vi "ERIO RT STATE Alarm.vi"(6 "Supervisory Variables In":T4={"Alarm Threshold"=0.0, "Shutdown"=FALSE, "Enable SNS Alarm"=FALSE, "Enable SNS Stage Notification"=FALSE, "Enable SQS Notification"=FALSE, "Enable S3 TDMS Signal Capture"=FALSE, "Enable SystemLink Signal Capture"=FALSE, "Capture Signal"=FALSE, "Server Update"=FALSE, "AWS Access Key"="AKIAINLDO2Y2PDFEWDOQ", "AWS Secret Key"="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", "Phone Number"="+15037066913", "Region"=enum."us-west-2", "AWS SQS Queue"="mynicloud-demotest2", "AWS S3 Bucket"="mynicloud-demotest2"}, 7 "RT State In":T1, 8 "error in (no error)":errorcluster, 9 "AWS Variables In":T6, 11 "EEISysLink.lvclass In":refnum<class "EEISysLink.lvclass">) -> (0 "error out":errorcluster, 1 "AWS Variables Out":T6, 3 "EEISysLink.lvclass Out":refnum<class "EEISysLink.lvclass">, 4 "Supervisory Variables Out":T4={"Alarm Threshold"=0.0, "Shutdown"=FALSE, "Enable SNS Alarm"=FALSE, "Enable SNS Stage Notification"=FALSE, "Enable SQS Notification"=FALSE, "Enable S3 TDMS Signal Capture"=FALSE, "Enable SystemLink Signal Capture"=FALSE, "Capture Signal"=FALSE, "Server Update"=FALSE, "AWS Access Key"="AKIAINLDO2Y2PDFEWDOQ", "AWS Secret Key"="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", "Phone Number"="+15037066913", "Region"=enum."us-west-2", "AWS SQS Queue"="mynicloud-demotest2", "AWS S3 Bucket"="mynicloud-demotest2"}, 5 "RT State Out":T1)   [LabVIEW 2017]
doc: "Execute the alarm state. Currently that means reporting the alarm in prescribed paths. \n\nJames Tillett P.E.\nEndeavor Engineering Inc.\nwww.endeavoreng.com"
uses:
  Class EEISysLink/EEISysLink.lvclass
  Controls/ERIO AWS Toolkit Variables.ctl
  <vilib>/AWS Toolkit/SQS/Queue/Queue.lvclass
  <vilib>/AWS Toolkit/SNS/Phone Number/Phone Number.lvclass
  <vilib>/AWS Toolkit/S3/Bucket/Bucket.lvclass
  Controls/ERIO Supervisory Variables.ctl
  <vilib>/AWS Toolkit/Core/HTTP Request/Region.ctl
  Controls/ERIO RT State Variables.ctl
  Controls/ERIO SystemStates.ctl
  Controls/ERIO Queue Data.ctl
  Controls/ERIO Worker Variables.ctl
  Controls/ERIO SoundOptions.ctl
  Class EEISysLink/Controls/SL Tag Scope.ctl
  <vilib>/AWS Toolkit/Core/HTTP Request/HTTP Request.lvclass
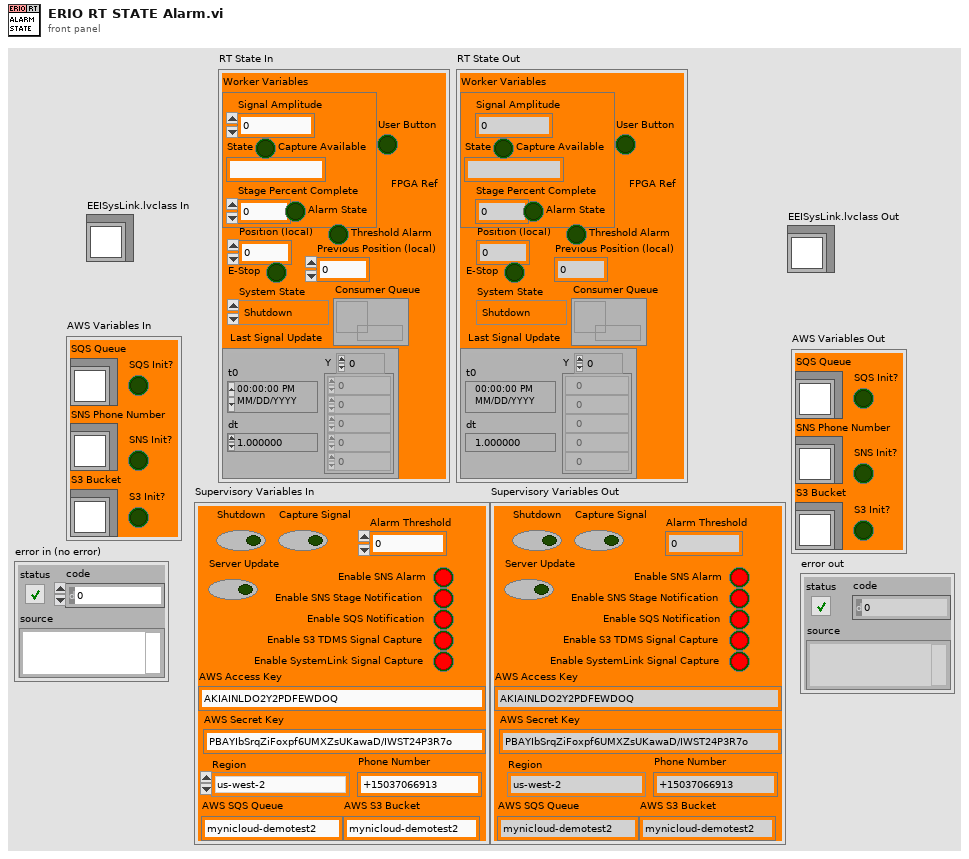
[diagram p1: front panel]
types:
  T1 = typedef "ERIO RT State Variables.ctl" = cluster{"Position (local)":i16, "E-Stop":bool, "System State":T2, "FPGA Ref":refnum<k20>, "Previous Position (local)":i16, "Consumer Queue":refnum<queue>, "Worker Variables":T3, "Threshold Alarm":bool, "User Button":bool, "Last Signal Update":waveform(dbl)}
  T2 = typedef "ERIO SystemStates.ctl" = enum16{"Shutdown", "E-STOP", "Reset Process", "Stage 1", "Stage 2", "Stage 3", "Alarm State"}
  T3 = typedef "ERIO Worker Variables.ctl" = cluster{"Signal Amplitude":dbl, "State":string, "Stage Percent Complete":dbl, "Alarm State":bool, "Capture Available":bool}
  T4 = typedef "ERIO Supervisory Variables.ctl" = cluster{"Alarm Threshold":dbl, "Shutdown":bool, "Enable SNS Alarm":bool, "Enable SNS Stage Notification":bool, "Enable SQS Notification":bool, "Enable S3 TDMS Signal Capture":bool, "Enable SystemLink Signal Capture":bool, "Capture Signal":bool, "Server Update":bool, "AWS Access Key":string, "AWS Secret Key":string, "Phone Number":string, "Region":T5, "AWS SQS Queue":string, "AWS S3 Bucket":string}
  T5 = typedef "NI_AWS_Core.lvlib/HTTP Request.lvclass/Region.ctl" = enum16{"us-east-1", "us-east-2", "us-west-1", "us-west-2", "ap-northeast-1", "ap-northeast-2", "ap-southeast-1", "ap-southeast-2", "ca-central-1", "eu-central-1", "eu-west-1", "eu-west-2", "sa-east-1"}
  T6 = typedef "ERIO AWS Toolkit Variables.ctl" = cluster{"SQS Queue":refnum<class "Queue.lvclass">, "SNS Phone Number":refnum<class "Phone Number.lvclass">, "S3 Bucket":refnum<class "Bucket.lvclass">, "SQS Init?":bool, "S3 Init?":bool, "SNS Init?":bool}
  T7 = typedef "EEISysLink.lvclass/SL Tag Scope.ctl" = enum16{"Local", "Server"}
  T8 = typedef "ERIO SoundOptions.ctl" = enum16{"Ding", "Boing", "Buzzer", "Horn"}
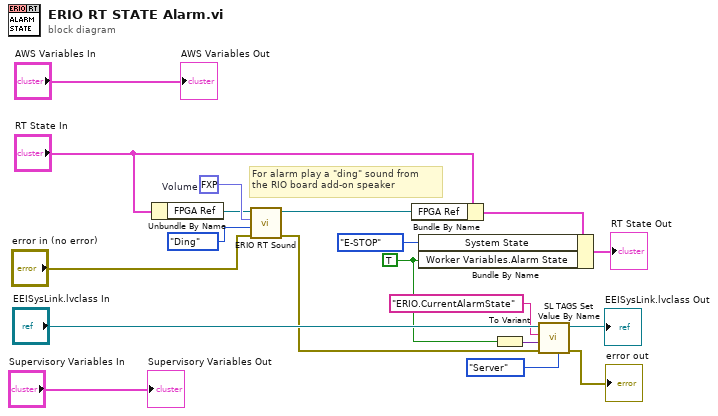
[diagram p0: block diagram]
diagram:
  w6 = TRUE ("Worker Variables.Alarm State")
  w19 = fxp<+/-,32,16> 5.0  # Volume
  # "For alarm play a \"ding\" sound from \nthe RIO board add-on speaker"
  n1 = Unbundle By Name("RT State In") -> ("FPGA Ref"=w16:refnum<k20>)
  n2 = call "ERIO RT Sound.vi"("error in"="error in (no error)", "Sound Options"=ERIO_SoundOptions."Ding" ("Enum"), "Volume"=w19, "FPGA VI Reference In"=w16) -> ("error out"=w4:errorcluster, "FPGA VI Reference Out"=w14:refnum<k20>)  [unwired: 6 in]
  n3 = Bundle By Name(cluster="RT State In", "FPGA Ref"=w14) -> (w13:T1)
  n4 = Bundle By Name(cluster=w13, "System State"=ERIO_SystemStates."E-STOP", "Worker Variables.Alarm State"=w6) -> (→"RT State Out":T1)
  n5 = To Variant(anything=w6) -> (Variant=w8:variant)
  n6 = call-dynamic "SL TAGS Set Value By Name.vi"("Tag Scope"=SL_Tag_Scope."Server", "error in (no error)"=w4, "Value"=w8, "Tag Name"="ERIO.CurrentAlarmState", "EEISysLink in"="EEISysLink.lvclass In") -> ("error out"=→"error out":errorcluster, "EEISysLink out"=→"EEISysLink.lvclass Out":refnum<class "EEISysLink.lvclass">)  [unwired: 5 in]
  "AWS Variables Out" <- "AWS Variables In"
  "Supervisory Variables Out" <- "Supervisory Variables In"
